vi "GetAzCamParameter.vi"(0 "Parameter":string) -> (1 "Error":bool, 2 "Value":string)   [LabVIEW 2014]
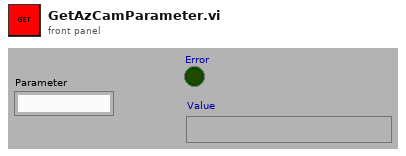
[diagram p1: front panel]
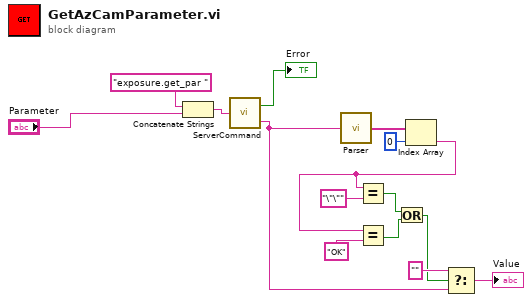
[diagram p0: block diagram]
diagram:
  n1 = Concatenate Strings("exposure.get_par " ("Attribute"), "Parameter") -> (w14:string)
  n2 = call "ServerCommand.vi"("Command"=w14) -> ("Error"=→"Error":bool, "Reply"=w7:string)
  n3 = call "Parser.vi"("string"=w7) -> ("Out Strings"=w11:string[])
  n4 = Index Array(array=w11, index=0) -> (element=w6:string)
  n5 = Equal?(x=w6, y="\"\"") -> (x = y?=w4:bool)
  n6 = Equal?(x=w6, y="OK") -> (x = y?=w3:bool)
  n7 = Or(x=w4, y=w3) -> (x .or. y?=w2:bool)
  n8 = Select(t="", s=w2, f=w7) -> (s? t:f=→"Value":string)
